vi "Unpack for gRPC.vi"(8 "error in":errorcluster, 9 "configuration / results":enum16{"Configuration", "Results"}(ring), 10 "any":T1, 11 "measurement customizations in":refnum<class "Measurement Plugin.lvclass">) -> (0 "error out":errorcluster, 2 "data value":variant, 3 "measurement customizations out":refnum<class "Measurement Plugin.lvclass">)   [LabVIEW 2021, in "Arbitrary Mode_PMIC.lvlib" / "Measurement Plugin.lvclass"]
uses:
  Measurement Plugin.lvclass
  Measurement Plugin.lvclass/Measurement Plugin.ctl
  Measurement Configuration.ctl
  Arbitrary Mode_PMIC.lvlib
  Measurement Results.ctl
  3ecd018e-d556-4cbc-bc60-c4ba57204520.vi
  a521b266-ce99-437c-923d-067dcf1e07fd.vi
  <vilib>/Plug-In SDKs/Measurements/Measurement Plugin Service/Measurement Plugin Service.lvclass
  C:/Program Files/National Instruments/LabVIEW 2021/vi.lib/Plug-In SDKs/Measurements/Measurement Plugin Service/Measurement Plugin Service.lvclass
  C:/pmic-labview/source/measurements/arbitrary mode/Arbitrary Mode_PMIC/Advanced/Measurement Plugin.lvclass
  <vilib>/gRPC/LabVIEW gRPC Library/Shared/Any.ctl
  <vilib>/gRPC/LabVIEW gRPC Library/grpc-lvsupport-release.lvlib
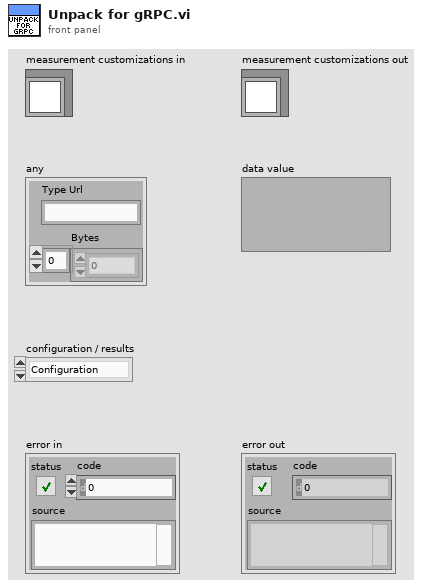
[diagram p1: front panel]
types:
  T1 = typedef "grpc-lvsupport-release.lvlib/Any.ctl" = cluster{"Type Url":string, "Bytes":u8[]}
  T2 = typedef "grpc-lvsupport-release.lvlib/grpcId.ctl" = u64
  T3 = typedef "Arbitrary Mode_PMIC.lvlib/Measurement Configuration.ctl" = cluster{"Source maximum power":dbl, "Source sample rate":dbl, "Source current limit":dbl, "Source resource name":string, "Source voltage pole-zero ratio":dbl, "Source voltage compensation frequency":dbl, "Source voltage gain bandwidth":dbl, "Source transient response":i32, "Set up voltage":dbl, "Trapezoid signal enable/disable":bool, "Trapezoid voltage delay t2":dbl, "Trapezoid voltage delay t1":dbl, "Trapezoid voltatge pulse duration":dbl, "Trapezoid voltage rising slew rate":dbl, "Trapezoid voltage falling slew rate":dbl, "Trapezoid voltage set point 2(V2)":dbl, "Trapezoid voltage set point 1(V1)":dbl, "Ramp signal enable/disable":bool, "Ramp voltage V1 time":dbl, "Ramp voltatge V2 time":dbl, "Ramp voltage ramp rate":dbl, "Ramp voltage set point 2(V2)":dbl, "Ramp voltage set point 1(V1)":dbl, "Source signal logging":u16[], "Source signal logging loop count":i64, "Source sense":i32, "Load enable/disable":bool, "Load resource name":string, "Load sense":i32, "Load voltage limit range":dbl, "Load current level range":dbl, "Load current level":dbl, "Load transient response":i32, "Load current gain bandwidth":dbl, "Load current compensation frequency":dbl, "Load current pole-zero ratio":dbl, "Scope enable/disable":bool, "Scope resource name":string, "Scope output channel name":string, "Scope sample rate":dbl, "Scope probe attenuation":dbl, "Scope vertical range":dbl, "Scope vertical coupling":enum32{"AC", "DC"}}
  T4 = typedef "Arbitrary Mode_PMIC.lvlib/Measurement Results.ctl" = cluster{"Source voltage dt":dbl, "Source voltages":dbl[], "Load voltage dt":dbl, "Load voltages":dbl[], "Scope amplitudes":dbl[], "Scope amplitude dt":dbl}
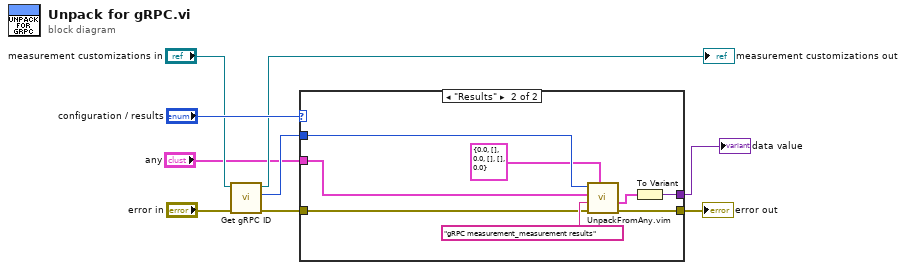
[diagram p0: block diagram]
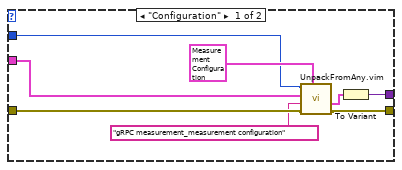
[diagram p2: hidden frame]
diagram:
  n1 = call <vilib>:"Get gRPC ID.vi"("error in"="error in", "measurement plugin service in"="measurement customizations in") -> ("error out"=w6:errorcluster, "gRPC ID"=w3:T2, "measurement plugin service out"=→"measurement customizations out":refnum<class "Measurement Plugin.lvclass">)  [unwired: 7 in]
  n2 = case shown="\"Results\"" "configuration / results" {
    tunnel: w6 -> [w15 w19]
    tunnel: "any" -> [w10 w18]
    tunnel: w3 -> [w12 w22]
    tunnel: [w16 w23] -> w9
    tunnel: [w17 w25] -> w1
    frame "Configuration" {
      n3 = call "UnpackFromAny.vim"("Data Type"=T3 {"Source maximum power"=1.2, "Source sample rate"=32.0, "Source current limit"=-32.0, "Source resource name"="Lorem ipsum dolor sit", "Source voltage pole-zero ratio"=1.0, "Source voltage compensation frequency"=1.0, "Source voltage gain bandwidth"=2000.0, "Source transient response"=1042, "Set up voltage"=0.0, "Trapezoid signal enable/disable"=TRUE, "Trapezoid voltage delay t2"=0.005, "Trapezoid voltage delay t1"=0.005, "Trapezoid voltatge pulse duration"=0.005, "Trapezoid voltage rising slew rate"=24.0, "Trapezoid voltage falling slew rate"=24.0, "Trapezoid voltage set point 2(V2)"=20.0, "Trapezoid voltage set point 1(V1)"=7.0, "Ramp signal enable/disable"=TRUE, "Ramp voltage V1 time"=0.005, "Ramp voltatge V2 time"=0.005, "Ramp voltage ramp rate"=6550.0, "Ramp voltage set point 2(V2)"=20.0, "Ramp voltage set point 1(V1)"=7.0, "Source signal logging"=[], "Source signal logging loop count"=1, "Source sense"=1009, "Load enable/disable"=TRUE, "Load resource name"="", "Load sense"=1009, "Load voltage limit range"=4.0, "Load current level range"=4.0, "Load current level"=0.03, "Load transient response"=1042, "Load current gain bandwidth"=14000.0, "Load current compensation frequency"=180000.0, "Load current pole-zero ratio"=0.3, "Scope enable/disable"=TRUE, "Scope resource name"="", "Scope output channel name"="0", "Scope sample rate"=1800000.0, "Scope probe attenuation"=1.0, "Scope vertical range"=10.0, "Scope vertical coupling"=enum."DC"} ("Measurement Configuration"), "error in"=w15, "Message Type"="gRPC measurement_measurement configuration", "Any"=w10, "gRPCid in"=w12) -> ("error out"=w16:errorcluster, "Unpacked Value"=w14:T3)  [unwired: 4 in, 1 out]
      n4 = To Variant(anything=w14) -> (Variant=w17:variant)
    }
    frame "Results" {
      n5 = call "UnpackFromAny.vim"("Data Type"=T4 {"Source voltage dt"=0.0, "Source voltages"=[], "Load voltage dt"=0.0, "Load voltages"=[], "Scope amplitudes"=[], "Scope amplitude dt"=0.0} ("Measurement Results"), "error in"=w19, "Message Type"="gRPC measurement_measurement results", "Any"=w18, "gRPCid in"=w22) -> ("error out"=w23:errorcluster, "Unpacked Value"=w24:T4)  [unwired: 4 in, 1 out]
      n6 = To Variant(anything=w24) -> (Variant=w25:variant)
    }
  }
  "error out" <- w9
  "data value" <- w1
